vi "App - analyze RUS V6.vi"() -> ()   [LabVIEW 2018] (continued)
"last mod"=timestamp(3493887848 s since 1904-01-01), "file name str"="D:\\Data\\Ultrasound\\LSCO\\LSCO22__130814c\\5_Cooling_2nd_try\\September_2014\\091814\\14.54900K_500_2500_2.10000V_0.00000T_Sep18-2014__08-24-08_001_091814.bin", "mod time(min)"=58231464.13333333, "file format"=enum."binary", "power(V)"=2.1, "Magn Field(T) "=0.0}, {"temperature"=14.546, "temperature str"="14.54600", "file path"=path "D:/Data/Ultrasound/LSCO/LSCO22__130814c/5_Cooling_2nd_try/September_2014/091814/14.54600K_500_2500_2.10000V_0.00000T_Sep18-2014__08-25-27_001_091814.bin", "last mod"=timestamp(3493887927 s since 1904-01-01), "file name str"="D:\\Data\\Ultrasound\\LSCO\\LSCO22__130814c\\5_Cooling_2nd_try\\September_2014\\091814\\14.54600K_500_2500_2.10000V_0.00000T_Sep18-2014__08-25-27_001_091814.bin", "mod time(min)"=58231465.45, "file format"=enum."binary", "power(V)"=2.1, "Magn Field(T) "=0.0}, {"temperature"=14.55, "temperature str"="14.55000", "file path"=path "D:/Data/Ultrasound/LSCO/LSCO22__130814c/5_Cooling_2nd_try/September_2014/091814/14.55000K_500_2500_2.10000V_0.00000T_Sep18-2014__08-26-47_001_091814.bin", "last mod"=timestamp(3493888007 s since 1904-01-01), "file name str"="D:\\Data\\Ultrasound\\LSCO\\LSCO22__130814c\\5_Cooling_2nd_try\\September_2014\\091814\\14.55000K_500_2500_2.10000V_0.00000T_Sep18-2014__08-26-47_001_091814.bin", "mod time(min)"=58231466.78333333, "file format"=enum."binary", "power(V)"=2.1, "Magn Field(T) "=0.0}, {"temperature"=14.556, "temperature str"="14.55600", "file path"=path "D:/Data/Ultrasound/LSCO/LSCO22__130814c/5_Cooling_2nd_try/September_2014/091814/14.55600K_500_2500_2.10000V_0.00000T_Sep18-2014__08-28-06_001_091814.bin", "last mod"=timestamp(3493888086 s since 1904-01-01), "file name str"="D:\\Data\\Ultrasound\\LSCO\\LSCO22__130814c\\5_Cooling_2nd_try\\September_2014\\091814\\14.55600K_500_2500_2.10000V_0.00000T_Sep18-2014__08-28-06_001_091814.bin", "mod time(min)"=58231468.1, "file format"=enum."binary", "power(V)"=2.1, "Magn Field(T) "=0.0}, {"temperature"=14.554, "temperature str"="14.55400", "file path"=path "D:/Data/Ultrasound/LSCO/LSCO22__130814c/5_Cooling_2nd_try/September_2014/091814/14.55400K_500_2500_2.10000V_0.00000T_Sep18-2014__08-29-25_001_091814.bin", "last mod"=timestamp(3493888165 s since 1904-01-01), "file name str"="D:\\Data\\Ultrasound\\LSCO\\LSCO22__130814c\\5_Cooling_2nd_try\\September_2014\\091814\\14.55400K_500_2500_2.10000V_0.00000T_Sep18-2014__08-29-25_001_091814.bin", "mod time(min)"=58231469.416666664, "file format"=enum."binary", "power(V)"=2.1, "Magn Field(T) "=0.0}, {"temperature"=14.553, "temperature str"="14.55300", "file path"=path "D:/Data/Ultrasound/LSCO/LSCO22__130814c/5_Cooling_2nd_try/September_2014/091814/14.55300K_500_2500_2.10000V_0.00000T_Sep18-2014__08-30-45_001_091814.bin", "last mod"=timestamp(3493888245 s since 1904-01-01), "file name str"="D:\\Data\\Ultrasound\\LSCO\\LSCO22__130814c\\5_Cooling_2nd_try\\September_2014\\091814\\14.55300K_500_2500_2.10000V_0.00000T_Sep18-2014__08-30-45_001_091814.bin", "mod time(min)"=58231470.75, "file format"=enum."binary", "power(V)"=2.1, "Magn Field(T) "=0.0}, {"temperature"=14.556, "temperature str"="14.55600", "file path"=path "D:/Data/Ultrasound/LSCO/LSCO22__130814c/5_Cooling_2nd_try/September_2014/091814/14.55600K_500_2500_2.10000V_0.00000T_Sep18-2014__08-32-04_001_091814.bin", "last mod"=timestamp(3493888324 s since 1904-01-01), "file name str"="D:\\Data\\Ultrasound\\LSCO\\LSCO22__130814c\\5_Cooling_2nd_try\\September_2014\\091814\\14.55600K_500_2500_2.10000V_0.00000T_Sep18-2014__08-32-04_001_091814.bin", "mod time(min)"=58231472.06666667, "file format"=enum."binary", "power(V)"=2.1, "Magn Field(T) "=0.0}, {"temperature"=14.556, "temperature str"="14.55600", "file path"=path "D:/Data/Ultrasound/LSCO/LSCO22__130814c/5_Cooling_2nd_try/September_2014/091814/14.55600K_500_2500_2.10000V_0.00000T_Sep18-2014__08-33-24_001_091814.bin", "last mod"=timestamp(3493888404 s since 1904-01-01), "file name str"="D:\\Data\\Ultrasound\\LSCO\\LSCO22__130814c\\5_Cooling_2nd_try\\September_2014\\091814\\14.55600K_500_2500_2.10000V_0.00000T_Sep18-2014__08-33-24_001_091814.bin", "mod time(min)"=58231473.4, "file format"=enum."binary", "power(V)"=2.1, "Magn Field(T) "=0.0}, {"temperature"=14.56, "temperature str"="14.56000", "file path"=path "D:/Data/Ultrasound/LSCO/LSCO22__130814c/5_Cooling_2nd_try/September_2014/091814/14.56000K_500_2500_2.10000V_0.00000T_Sep18-2014__08-34-43_001_091814.bin", "last mod"=timestamp(3493888483 s since 1904-01-01), "file name str"="D:\\Data\\Ultrasound\\LSCO\\LSCO22__130814c\\5_Cooling_2nd_try\\September_2014\\091814\\14.56000K_500_2500_2.10000V_0.00000T_Sep18-2014__08-34-43_001_091814.bin", "mod time(min)"=58231474.71666667, "file format"=enum."binary", "power(V)"=2.1, "Magn Field(T) "=0.0}, {"temperature"=14.56, "temperature str"="14.56000", "file path"=path "D:/Data/Ultrasound/LSCO/LSCO22__130814c/5_Cooling_2nd_try/September_2014/091814/14.56000K_500_2500_2.10000V_0.00000T_Sep18-2014__08-36-02_001_091814.bin", "last mod"=timestamp(3493888562 s since 1904-01-01), "file name str"="D:\\Data\\Ultrasound\\LSCO\\LSCO22__130814c\\5_Cooling_2nd_try\\September_2014\\091814\\14.56000K_500_2500_2.10000V_0.00000T_Sep18-2014__08-36-02_001_091814.bin", "mod time(min)"=58231476.03333333, "file format"=enum."binary", "power(V)"=2.1, "Magn Field(T) "=0.0}, {"temperature"=14.561, "temperature str"="14.56100", "file path"=path "D:/Data/Ultrasound/LSCO/LSCO22__130814c/5_Cooling_2nd_try/September_2014/091814/14.56100K_500_2500_2.10000V_0.00000T_Sep18-2014__08-37-22_001_091814.bin", "last mod"=timestamp(3493888642 s since 1904-01-01), "file name str"="D:\\Data\\Ultrasound\\LSCO\\LSCO22__130814c\\5_Cooling_2nd_try\\September_2014\\091814\\14.56100K_500_2500_2.10000V_0.00000T_Sep18-2014__08-37-22_001_091814.bin", "mod time(min)"=58231477.36666667, "file format"=enum."binary", "power(V)"=2.1, "Magn Field(T) "=0.0}, {"temperature"=14.562, "temperature str"="14.56200", "file path"=path "D:/Data/Ultrasound/LSCO/LSCO22__130814c/5_Cooling_2nd_try/September_2014/091814/14.56200K_500_2500_2.10000V_0.00000T_Sep18-2014__08-38-41_001_091814.bin", "last mod"=timestamp(3493888721 s since 1904-01-01), "file name str"="D:\\Data\\Ultrasound\\LSCO\\LSCO22__130814c\\5_Cooling_2nd_try\\September_2014\\091814\\14.56200K_500_2500_2.10000V_0.00000T_Sep18-2014__08-38-41_001_091814.bin", "mod time(min)"=58231478.68333333, "file format"=enum."binary", "power(V)"=2.1, "Magn Field(T) "=0.0}, {"temperature"=14.56, "temperature str"="14.56000", "file path"=path "D:/Data/Ultrasound/LSCO/LSCO22__130814c/5_Cooling_2nd_try/September_2014/091814/14.56000K_500_2500_2.10000V_0.00000T_Sep18-2014__08-40-00_001_091814.bin", "last mod"=timestamp(3493888800 s since 1904-01-01), "file name str"="D:\\Data\\Ultrasound\\LSCO\\LSCO22__130814c\\5_Cooling_2nd_try\\September_2014\\091814\\14.56000K_500_2500_2.10000V_0.00000T_Sep18-2014__08-40-00_001_091814.bin", "mod time(min)"=58231480.0, "file format"=enum."binary", "power(V)"=2.1, "Magn Field(T) "=0.0}, {"temperature"=14.56, "temperature str"="14.56000", "file path"=path "D:/Data/Ultrasound/LSCO/LSCO22__130814c/5_Cooling_2nd_try/September_2014/091814/14.56000K_500_2500_2.10000V_0.00000T_Sep18-2014__08-41-20_001_091814.bin", "last mod"=timestamp(3493888880 s since 1904-01-01), "file name str"="D:\\Data\\Ultrasound\\LSCO\\LSCO22__130814c\\5_Cooling_2nd_try\\September_2014\\091814\\14.56000K_500_2500_2.10000V_0.00000T_Sep18-2014__08-41-20_001_091814.bin", "mod time(min)"=58231481.333333336, "file format"=enum."binary", "power(V)"=2.1, "Magn Field(T) "=0.0}, {"temperature"=14.561, "temperature str"="14.56100", "file path"=path "D:/Data/Ultrasound/LSCO/LSCO22__130814c/5_Cooling_2nd_try/September_2014/091814/14.56100K_500_2500_2.10000V_0.00000T_Sep18-2014__08-42-39_001_091814.bin", "last mod"=timestamp(3493888959 s since 1904-01-01), "file name str"="D:\\Data\\Ultrasound\\LSCO\\LSCO22__130814c\\5_Cooling_2nd_try\\September_2014\\091814\\14.56100K_500_2500_2.10000V_0.00000T_Sep18-2014__08-42-39_001_091814.bin", "mod time(min)"=58231482.65, "file format"=enum."binary", "power(V)"=2.1, "Magn Field(T) "=0.0}, {"temperature"=14.563, "temperature str"="14.56300", "file path"=path "D:/Data/Ultrasound/LSCO/LSCO22__130814c/5_Cooling_2nd_try/September_2014/091814/14.56300K_500_2500_2.10000V_0.00000T_Sep18-2014__08-43-59_001_091814.bin", "last mod"=timestamp(3493889039 s since 1904-01-01), "file name str"="D:\\Data\\Ultrasound\\LSCO\\LSCO22__130814c\\5_Cooling_2nd_try\\September_2014\\091814\\14.56300K_500_2500_2.10000V_0.00000T_Sep18-2014__08-43-59_001_091814.bin", "mod time(min)"=58231483.983333334, "file format"=enum."binary", "power(V)"=2.1, "Magn Field(T) "=0.0}, {"temperature"=14.564, "temperature str"="14.56400", "file path"=path "D:/Data/Ultrasound/LSCO/LSCO22__130814c/5_Cooling_2nd_try/September_2014/091814/14.56400K_500_2500_2.10000V_0.00000T_Sep18-2014__08-45-18_001_091814.bin", "last mod"=timestamp(3493889118 s since 1904-01-01), "file name str"="D:\\Data\\Ultrasound\\LSCO\\LSCO22__130814c\\5_Cooling_2nd_try\\September_2014\\091814\\14.56400K_500_2500_2.10000V_0.00000T_Sep18-2014__08-45-18_001_091814.bin", "mod time(min)"=58231485.3, "file format"=enum."binary", "power(V)"=2.1, "Magn Field(T) "=0.0}, {"temperature"=14.572, "temperature str"="14.57200", "file path"=path "D:/Data/Ultrasound/LSCO/LSCO22__130814c/5_Cooling_2nd_try/September_2014/091814/14.57200K_500_2500_2.10000V_0.00000T_Sep18-2014__08-46-37_001_091814.bin", "last mod"=timestamp(3493889197 s since 1904-01-01), "file name str"="D:\\Data\\Ultrasound\\LSCO\\LSCO22__130814c\\5_Cooling_2nd_try\\September_2014\\091814\\14.57200K_500_2500_2.10000V_0.00000T_Sep18-2014__08-46-37_001_091814.bin", "mod time(min)"=58231486.61666667, "file format"=enum."binary", "power(V)"=2.1, "Magn Field(T) "=0.0}, {"temperature"=14.568, "temperature str"="14.56800", "file path"=path "D:/Data/Ultrasound/LSCO/LSCO22__130814c/5_Cooling_2nd_try/September_2014/091814/14.56800K_500_2500_2.10000V_0.00000T_Sep18-2014__08-47-57_001_091814.bin", "last mod"=timestamp(3493889277 s since 1904-01-01), "file name str"="D:\\Data\\Ultrasound\\LSCO\\LSCO22__130814c\\5_Cooling_2nd_try\\September_2014\\091814\\14.56800K_500_2500_2.10000V_0.00000T_Sep18-2014__08-47-57_001_091814.bin", "mod time(min)"=58231487.95, "file format"=enum."binary", "power(V)"=2.1, "Magn Field(T) "=0.0}, {"temperature"=14.565, "temperature str"="14.56500", "file path"=path "D:/Data/Ultrasound/LSCO/LSCO22__130814c/5_Cooling_2nd_try/September_2014/091814/14.56500K_500_2500_2.10000V_0.00000T_Sep18-2014__08-49-16_001_091814.bin", "last mod"=timestamp(3493889356 s since 1904-01-01), "file name str"="D:\\Data\\Ultrasound\\LSCO\\LSCO22__130814c\\5_Cooling_2nd_try\\September_2014\\091814\\14.56500K_500_2500_2.10000V_0.00000T_Sep18-2014__08-49-16_001_091814.bin", "mod time(min)"=58231489.266666666, "file format"=enum."binary", "power(V)"=2.1, "Magn Field(T) "=0.0}, {"temperature"=14.569, "temperature str"="14.56900", "file path"=path "D:/Data/Ultrasound/LSCO/LSCO22__130814c/5_Cooling_2nd_try/September_2014/091814/14.56900K_500_2500_2.10000V_0.00000T_Sep18-2014__08-50-36_001_091814.bin", "last mod"=timestamp(3493889436 s since 1904-01-01), "file name str"="D:\\Data\\Ultrasound\\LSCO\\LSCO22__130814c\\5_Cooling_2nd_try\\September_2014\\091814\\14.56900K_500_2500_2.10000V_0.00000T_Sep18-2014__08-50-36_001_091814.bin", "mod time(min)"=58231490.6, "file format"=enum."binary", "power(V)"=2.1, "Magn Field(T) "=0.0}, {"temperature"=14.577, "temperature str"="14.57700", "file path"=path "D:/Data/Ultrasound/LSCO/LSCO22__130814c/5_Cooling_2nd_try/September_2014/091814/14.57700K_500_2500_2.10000V_0.00000T_Sep18-2014__08-51-55_001_091814.bin", "last mod"=timestamp(3493889515 s since 1904-01-01), "file name str"="D:\\Data\\Ultrasound\\LSCO\\LSCO22__130814c\\5_Cooling_2nd_try\\September_2014\\091814\\14.57700K_500_2500_2.10000V_0.00000T_Sep18-2014__08-51-55_001_091814.bin", "mod time(min)"=58231491.916666664, "file format"=enum."binary", "power(V)"=2.1, "Magn Field(T) "=0.0}, {"temperature"=14.571, "temperature str"="14.57100", "file path"=path "D:/Data/Ultrasound/LSCO/LSCO22__130814c/5_Cooling_2nd_try/September_2014/091814/14.57100K_500_2500_2.10000V_0.00000T_Sep18-2014__08-53-14_001_091814.bin", "last mod"=timestamp(3493889594 s since 1904-01-01), "file name str"="D:\\Data\\Ultrasound\\LSCO\\LSCO22__130814c\\5_Cooling_2nd_try\\September_2014\\091814\\14.57100K_500_2500_2.10000V_0.00000T_Sep18-2014__08-53-14_001_091814.bin", "mod time(min)"=58231493.233333334, "file format"=enum."binary", "power(V)"=2.1, "Magn Field(T) "=0.0}, {"temperature"=14.58, "temperature str"="14.58000", "file path"=path "D:/Data/Ultrasound/LSCO/LSCO22__130814c/5_Cooling_2nd_try/September_2014/091814/14.58000K_500_2500_2.10000V_0.00000T_Sep18-2014__08-54-34_001_091814.bin", "last mod"=timestamp(3493889674 s since 1904-01-01), "file name str"="D:\\Data\\Ultrasound\\LSCO\\LSCO22__130814c\\5_Cooling_2nd_try\\September_2014\\091814\\14.58000K_500_2500_2.10000V_0.00000T_Sep18-2014__08-54-34_001_091814.bin", "mod time(min)"=58231494.56666667, "file format"=enum."binary", "power(V)"=2.1, "Magn Field(T) "=0.0}, {"temperature"=14.578, "temperature str"="14.57800", "file path"=path "D:/Data/Ultrasound/LSCO/LSCO22__130814c/5_Cooling_2nd_try/September_2014/091814/14.57800K_500_2500_2.10000V_0.00000T_Sep18-2014__08-55-53_001_091814.bin", "last mod"=timestamp(3493889753 s since 1904-01-01), "file name str"="D:\\Data\\Ultrasound\\LSCO\\LSCO22__130814c\\5_Cooling_2nd_try\\September_2014\\091814\\14.57800K_500_2500_2.10000V_0.00000T_Sep18-2014__08-55-53_001_091814.bin", "mod time(min)"=58231495.88333333, "file format"=enum."binary", "power(V)"=2.1, "Magn Field(T) "=0.0}, {"temperature"=14.579, "temperature str"="14.57900", "file path"=path "D:/Data/Ultrasound/LSCO/LSCO22__130814c/5_Cooling_2nd_try/September_2014/091814/14.57900K_500_2500_2.10000V_0.00000T_Sep18-2014__08-57-12_001_091814.bin", "last mod"=timestamp(3493889832 s since 1904-01-01), "file name str"="D:\\Data\\Ultrasound\\LSCO\\LSCO22__130814c\\5_Cooling_2nd_try\\September_2014\\091814\\14.57900K_500_2500_2.10000V_0.00000T_Sep18-2014__08-57-12_001_091814.bin", "mod time(min)"=58231497.2, "file format"=enum."binary", "power(V)"=2.1, "Magn Field(T) "=0.0}, {"temperature"=14.581, "temperature str"="14.58100", "file path"=path "D:/Data/Ultrasound/LSCO/LSCO22__130814c/5_Cooling_2nd_try/September_2014/091814/14.58100K_500_2500_2.10000V_0.00000T_Sep18-2014__08-58-31_001_091814.bin", "last mod"=timestamp(3493889911 s since 1904-01-01), "file name str"="D:\\Data\\Ultrasound\\LSCO\\LSCO22__130814c\\5_Cooling_2nd_try\\September_2014\\091814\\14.58100K_500_2500_2.10000V_0.00000T_Sep18-2014__08-58-31_001_091814.bin", "mod time(min)"=58231498.516666666, "file format"=enum."binary", "power(V)"=2.1, "Magn Field(T) "=0.0}, {"temperature"=14.58, "temperature str"="14.58000", "file path"=path "D:/Data/Ultrasound/LSCO/LSCO22__130814c/5_Cooling_2nd_try/September_2014/091814/14.58000K_500_2500_2.10000V_0.00000T_Sep18-2014__08-59-50_001_091814.bin", "last mod"=timestamp(3493889990 s since 1904-01-01), "file name str"="D:\\Data\\Ultrasound\\LSCO\\LSCO22__130814c\\5_Cooling_2nd_try\\September_2014\\091814\\14.58000K_500_2500_2.10000V_0.00000T_Sep18-2014__08-59-50_001_091814.bin", "mod time(min)"=58231499.833333336, "file format"=enum."binary", "power(V)"=2.1, "Magn Field(T) "=0.0}, {"temperature"=14.577, "temperature str"="14.57700", "file path"=path "D:/Data/Ultrasound/LSCO/LSCO22__130814c/5_Cooling_2nd_try/September_2014/091814/14.57700K_500_2500_2.10000V_0.00000T_Sep18-2014__09-01-10_001_091814.bin", "last mod"=timestamp(3493890070 s since 1904-01-01), "file name str"="D:\\Data\\Ultrasound\\LSCO\\LSCO22__130814c\\5_Cooling_2nd_try\\September_2014\\091814\\14.57700K_500_2500_2.10000V_0.00000T_Sep18-2014__09-01-10_001_091814.bin", "mod time(min)"=58231501.166666664, "file format"=enum."binary", "power(V)"=2.1, "Magn Field(T) "=0.0}, {"temperature"=14.58, "temperature str"="14.58000", "file path"=path "D:/Data/Ultrasound/LSCO/LSCO22__130814c/5_Cooling_2nd_try/September_2014/091814/14.58000K_500_2500_2.10000V_0.00000T_Sep18-2014__09-02-29_001_091814.bin", "last mod"=timestamp(3493890149 s since 1904-01-01), "file name str"="D:\\Data\\Ultrasound\\LSCO\\LSCO22__130814c\\5_Cooling_2nd_try\\September_2014\\091814\\14.58000K_500_2500_2.10000V_0.00000T_Sep18-2014__09-02-29_001_091814.bin", "mod time(min)"=58231502.483333334, "file format"=enum."binary", "power(V)"=2.1, "Magn Field(T) "=0.0}, {"temperature"=14.583, "temperature str"="14.58300", "file path"=path "D:/Data/Ultrasound/LSCO/LSCO22__130814c/5_Cooling_2nd_try/September_2014/091814/14.58300K_500_2500_2.10000V_0.00000T_Sep18-2014__09-03-48_001_091814.bin", "last mod"=timestamp(3493890228 s since 1904-01-01), "file name str"="D:\\Data\\Ultrasound\\LSCO\\LSCO22__130814c\\5_Cooling_2nd_try\\September_2014\\091814\\14.58300K_500_2500_2.10000V_0.00000T_Sep18-2014__09-03-48_001_091814.bin", "mod time(min)"=58231503.8, "file format"=enum."binary", "power(V)"=2.1, "Magn Field(T) "=0.0}, {"temperature"=14.582, "temperature str"="14.58200", "file path"=path "D:/Data/Ultrasound/LSCO/LSCO22__130814c/5_Cooling_2nd_try/September_2014/091814/14.58200K_500_2500_2.10000V_0.00000T_Sep18-2014__09-05-08_001_091814.bin", "last mod"=timestamp(3493890308 s since 1904-01-01), "file name str"="D:\\Data\\Ultrasound\\LSCO\\LSCO22__130814c\\5_Cooling_2nd_try\\September_2014\\091814\\14.58200K_500_2500_2.10000V_0.00000T_Sep18-2014__09-05-08_001_091814.bin", "mod time(min)"=58231505.13333333, "file format"=enum."binary", "power(V)"=2.1, "Magn Field(T) "=0.0}, {"temperature"=14.584, "temperature str"="14.58400", "file path"=path "D:/Data/Ultrasound/LSCO/LSCO22__130814c/5_Cooling_2nd_try/September_2014/091814/14.58400K_500_2500_2.10000V_0.00000T_Sep18-2014__09-06-27_001_091814.bin", "last mod"=timestamp(3493890387 s since 1904-01-01), "file name str"="D:\\Data\\Ultrasound\\LSCO\\LSCO22__130814c\\5_Cooling_2nd_try\\September_2014\\091814\\14.58400K_500_2500_2.10000V_0.00000T_Sep18-2014__09-06-27_001_091814.bin", "mod time(min)"=58231506.45, "file format"=enum."binary", "power(V)"=2.1, "Magn Field(T) "=0.0}, {"temperature"=14.584, "temperature str"="14.58400", "file path"=path "D:/Data/Ultrasound/LSCO/LSCO22__130814c/5_Cooling_2nd_try/September_2014/091814/14.58400K_500_2500_2.10000V_0.00000T_Sep18-2014__09-07-46_001_091814.bin", "last mod"=timestamp(3493890466 s since 1904-01-01), "file name str"="D:\\Data\\Ultrasound\\LSCO\\LSCO22__130814c\\5_Cooling_2nd_try\\September_2014\\091814\\14.58400K_500_2500_2.10000V_0.00000T_Sep18-2014__09-07-46_001_091814.bin", "mod time(min)"=58231507.766666666, "file format"=enum."binary", "power(V)"=2.1, "Magn Field(T) "=0.0}, {"temperature"=14.585, "temperature str"="14.58500", "file path"=path "D:/Data/Ultrasound/LSCO/LSCO22__130814c/5_Cooling_2nd_try/September_2014/091814/14.58500K_500_2500_2.10000V_0.00000T_Sep18-2014__09-09-06_001_091814.bin", "last mod"=timestamp(3493890546 s since 1904-01-01), "file name str"="D:\\Data\\Ultrasound\\LSCO\\LSCO22__130814c\\5_Cooling_2nd_try\\September_2014\\091814\\14.58500K_500_2500_2.10000V_0.00000T_Sep18-2014__09-09-06_001_091814.bin", "mod time(min)"=58231509.1, "file format"=enum."binary", "power(V)"=2.1, "Magn Field(T) "=0.0}, {"temperature"=14.585, "temperature str"="14.58500", "file path"=path "D:/Data/Ultrasound/LSCO/LSCO22__130814c/5_Cooling_2nd_try/September_2014/091814/14.58500K_500_2500_2.10000V_0.00000T_Sep18-2014__09-10-25_001_091814.bin", "last mod"=timestamp(3493890625 s since 1904-01-01), "file name str"="D:\\Data\\Ultrasound\\LSCO\\LSCO22__130814c\\5_Cooling_2nd_try\\September_2014\\091814\\14.58500K_500_2500_2.10000V_0.00000T_Sep18-2014__09-10-25_001_091814.bin", "mod time(min)"=58231510.416666664, "file format"=enum."binary", "power(V)"=2.1, "Magn Field(T) "=0.0}, {"temperature"=14.585, "temperature str"="14.58500", "file path"=path "D:/Data/Ultrasound/LSCO/LSCO22__130814c/5_Cooling_2nd_try/September_2014/091814/14.58500K_500_2500_2.10000V_0.00000T_Sep18-2014__09-11-44_001_091814.bin", "last mod"=timestamp(3493890704 s since 1904-01-01), "file name str"="D:\\Data\\Ultrasound\\LSCO\\LSCO22__130814c\\5_Cooling_2nd_try\\September_2014\\091814\\14.58500K_500_2500_2.10000V_0.00000T_Sep18-2014__09-11-44_001_091814.bin", "mod time(min)"=58231511.733333334, "file format"=enum."binary", "power(V)"=2.1, "Magn Field(T) "=0.0}, {"temperature"=14.585, "temperature str"="14.58500", "file path"=path "D:/Data/Ultrasound/LSCO/LSCO22__130814c/5_Cooling_2nd_try/September_2014/091814/14.58500K_500_2500_2.10000V_0.00000T_Sep18-2014__09-13-04_001_091814.bin", "last mod"=timestamp(3493890784 s since 1904-01-01), "file name str"="D:\\Data\\Ultrasound\\LSCO\\LSCO22__130814c\\5_Cooling_2nd_try\\September_2014\\091814\\14.58500K_500_2500_2.10000V_0.00000T_Sep18-2014__09-13-04_001_091814.bin", "mod time(min)"=58231513.06666667, "file format"=enum."binary", "power(V)"=2.1, "Magn Field(T) "=0.0}, {"temperature"=14.587, "temperature str"="14.58700", "file path"=path "D:/Data/Ultrasound/LSCO/LSCO22__130814c/5_Cooling_2nd_try/September_2014/091814/14.58700K_500_2500_2.10000V_0.00000T_Sep18-2014__09-14-23_001_091814.bin", "last mod"=timestamp(3493890863 s since 1904-01-01), "file name str"="D:\\Data\\Ultrasound\\LSCO\\LSCO22__130814c\\5_Cooling_2nd_try\\September_2014\\091814\\14.58700K_500_2500_2.10000V_0.00000T_Sep18-2014__09-14-23_001_091814.bin", "mod time(min)"=58231514.38333333, "file format"=enum."binary", "power(V)"=2.1, "Magn Field(T) "=0.0}, {"temperature"=14.593, "temperature str"="14.59300", "file path"=path "D:/Data/Ultrasound/LSCO/LSCO22__130814c/5_Cooling_2nd_try/September_2014/091814/14.59300K_500_2500_2.10000V_0.00000T_Sep18-2014__09-15-43_001_091814.bin", "last mod"=timestamp(3493890943 s since 1904-01-01), "file name str"="D:\\Data\\Ultrasound\\LSCO\\LSCO22__130814c\\5_Cooling_2nd_try\\September_2014\\091814\\14.59300K_500_2500_2.10000V_0.00000T_Sep18-2014__09-15-43_001_091814.bin", "mod time(min)"=58231515.71666667, "file format"=enum."binary", "power(V)"=2.1, "Magn Field(T) "=0.0}, {"temperature"=14.595, "temperature str"="14.59500", "file path"=path "D:/Data/Ultrasound/LSCO/LSCO22__130814c/5_Cooling_2nd_try/September_2014/091814/14.59500K_500_2500_2.10000V_0.00000T_Sep18-2014__09-17-02_001_091814.bin", "last mod"=timestamp(3493891022 s since 1904-01-01), "file name str"="D:\\Data\\Ultrasound\\LSCO\\LSCO22__130814c\\5_Cooling_2nd_try\\September_2014\\091814\\14.59500K_500_2500_2.10000V_0.00000T_Sep18-2014__09-17-02_001_091814.bin", "mod time(min)"=58231517.03333333, "file format"=enum."binary", "power(V)"=2.1, "Magn Field(T) "=0.0}, {"temperature"=14.597, "temperature str"="14.59700", "file path"=path "D:/Data/Ultrasound/LSCO/LSCO22__130814c/5_Cooling_2nd_try/September_2014/091814/14.59700K_500_2500_2.10000V_0.00000T_Sep18-2014__09-18-21_001_091814.bin", "last mod"=timestamp(3493891101 s since 1904-01-01), "file name str"="D:\\Data\\Ultrasound\\LSCO\\LSCO22__130814c\\5_Cooling_2nd_try\\September_2014\\091814\\14.59700K_500_2500_2.10000V_0.00000T_Sep18-2014__09-18-21_001_091814.bin", "mod time(min)"=58231518.35, "file format"=enum."binary", "power(V)"=2.1, "Magn Field(T) "=0.0}, {"temperature"=14.595, "temperature str"="14.59500", "file path"=path "D:/Data/Ultrasound/LSCO/LSCO22__130814c/5_Cooling_2nd_try/September_2014/091814/14.59500K_500_2500_2.10000V_0.00000T_Sep18-2014__09-19-41_001_091814.bin", "last mod"=timestamp(3493891181 s since 1904-01-01), "file name str"="D:\\Data\\Ultrasound\\LSCO\\LSCO22__130814c\\5_Cooling_2nd_try\\September_2014\\091814\\14.59500K_500_2500_2.10000V_0.00000T_Sep18-2014__09-19-41_001_091814.bin", "mod time(min)"=58231519.68333333, "file format"=enum."binary", "power(V)"=2.1, "Magn Field(T) "=0.0}, {"temperature"=14.597, "temperature str"="14.59700", "file path"=path "D:/Data/Ultrasound/LSCO/LSCO22__130814c/5_Cooling_2nd_try/September_2014/091814/14.59700K_500_2500_2.10000V_0.00000T_Sep18-2014__09-21-00_001_091814.bin", "last mod"=timestamp(3493891260 s since 1904-01-01), "file name str"="D:\\Data\\Ultrasound\\LSCO\\LSCO22__130814c\\5_Cooling_2nd_try\\September_2014\\091814\\14.59700K_500_2500_2.10000V_0.00000T_Sep18-2014__09-21-00_001_091814.bin", "mod time(min)"=58231521.0, "file format"=enum."binary", "power(V)"=2.1, "Magn Field(T) "=0.0}, {"temperature"=14.595, "temperature str"="14.59500", "file path"=path "D:/Data/Ultrasound/LSCO/LSCO22__130814c/5_Cooling_2nd_try/September_2014/091814/14.59500K_500_2500_2.10000V_0.00000T_Sep18-2014__09-22-19_001_091814.bin", "last mod"=timestamp(3493891339 s since 1904-01-01), "file name str"="D:\\Data\\Ultrasound\\LSCO\\LSCO22__130814c\\5_Cooling_2nd_try\\September_2014\\091814\\14.59500K_500_2500_2.10000V_0.00000T_Sep18-2014__09-22-19_001_091814.bin", "mod time(min)"=58231522.31666667, "file format"=enum."binary", "power(V)"=2.1, "Magn Field(T) "=0.0}, {"temperature"=14.597, "temperature str"="14.59700", "file path"=path "D:/Data/Ultrasound/LSCO/LSCO22__130814c/5_Cooling_2nd_try/September_2014/091814/14.59700K_500_2500_2.10000V_0.00000T_Sep18-2014__09-23-39_001_091814.bin", "last mod"=timestamp(3493891419 s since 1904-01-01), "file name str"="D:\\Data\\Ultrasound\\LSCO\\LSCO22__130814c\\5_Cooling_2nd_try\\September_2014\\091814\\14.59700K_500_2500_2.10000V_0.00000T_Sep18-2014__09-23-39_001_091814.bin", "mod time(min)"=58231523.65, "file format"=enum."binary", "power(V)"=2.1, "Magn Field(T) "=0.0}, {"temperature"=14.597, "temperature str"="14.59700", "file path"=path "D:/Data/Ultrasound/LSCO/LSCO22__130814c/5_Cooling_2nd_try/September_2014/091814/14.59700K_500_2500_2.10000V_0.00000T_Sep18-2014__09-24-58_001_091814.bin", "last mod"=timestamp(3493891498 s since 1904-01-01), "file name str"="D:\\Data\\Ultrasound\\LSCO\\LSCO22__130814c\\5_Cooling_2nd_try\\September_2014\\091814\\14.59700K_500_2500_2.10000V_0.00000T_Sep18-2014__09-24-58_001_091814.bin", "mod time(min)"=58231524.96666667, "file format"=enum."binary", "power(V)"=2.1, "Magn Field(T) "=0.0}, {"temperature"=14.599, "temperature str"="14.59900", "file path"=path "D:/Data/Ultrasound/LSCO/LSCO22__130814c/5_Cooling_2nd_try/September_2014/091814/14.59900K_500_2500_2.10000V_0.00000T_Sep18-2014__09-26-18_001_091814.bin", "last mod"=timestamp(3493891578 s since 1904-01-01), "file name str"="D:\\Data\\Ultrasound\\LSCO\\LSCO22__130814c\\5_Cooling_2nd_try\\September_2014\\091814\\14.59900K_500_2500_2.10000V_0.00000T_Sep18-2014__09-26-18_001_091814.bin", "mod time(min)"=58231526.3, "file format"=enum."binary", "power(V)"=2.1, "Magn Field(T) "=0.0}, {"temperature"=14.599, "temperature str"="14.59900", "file path"=path "D:/Data/Ultrasound/LSCO/LSCO22__130814c/5_Cooling_2nd_try/September_2014/091814/14.59900K_500_2500_2.10000V_0.00000T_Sep18-2014__09-27-37_001_091814.bin", "last mod"=timestamp(3493891657 s since 1904-01-01), "file name str"="D:\\Data\\Ultrasound\\LSCO\\LSCO22__130814c\\5_Cooling_2nd_try\\September_2014\\091814\\14.59900K_500_2500_2.10000V_0.00000T_Sep18-2014__09-27-37_001_091814.bin", "mod time(min)"=58231527.61666667, "file format"=enum."binary", "power(V)"=2.1, "Magn Field(T) "=0.0}, {"temperature"=14.599, "temperature str"="14.59900", "file path"=path "D:/Data/Ultrasound/LSCO/LSCO22__130814c/5_Cooling_2nd_try/September_2014/091814/14.59900K_500_2500_2.10000V_0.00000T_Sep18-2014__09-28-56_001_091814.bin", "last mod"=timestamp(3493891736 s since 1904-01-01), "file name str"="D:\\Data\\Ultrasound\\LSCO\\LSCO22__130814c\\5_Cooling_2nd_try\\September_2014\\091814\\14.59900K_500_2500_2.10000V_0.00000T_Sep18-2014__09-28-56_001_091814.bin", "mod time(min)"=58231528.93333333, "file format"=enum."binary", "power(V)"=2.1, "Magn Field(T) "=0.0}, {"temperature"=14.601, "temperature str"="14.60100", "file path"=path "D:/Data/Ultrasound/LSCO/LSCO22__130814c/5_Cooling_2nd_try/September_2014/091814/14.60100K_500_2500_2.10000V_0.00000T_Sep18-2014__09-30-16_001_091814.bin", "last mod"=timestamp(3493891816 s since 1904-01-01), "file name str"="D:\\Data\\Ultrasound\\LSCO\\LSCO22__130814c\\5_Cooling_2nd_try\\September_2014\\091814\\14.60100K_500_2500_2.10000V_0.00000T_Sep18-2014__09-30-16_001_091814.bin", "mod time(min)"=58231530.266666666, "file format"=enum."binary", "power(V)"=2.1, "Magn Field(T) "=0.0}, {"temperature"=14.605, "temperature str"="14.60500", "file path"=path "D:/Data/Ultrasound/LSCO/LSCO22__130814c/5_Cooling_2nd_try/September_2014/091814/14.60500K_500_2500_2.10000V_0.00000T_Sep18-2014__09-31-35_001_091814.bin", "last mod"=timestamp(3493891895 s since 1904-01-01), "file name str"="D:\\Data\\Ultrasound\\LSCO\\LSCO22__130814c\\5_Cooling_2nd_try\\September_2014\\091814\\14.60500K_500_2500_2.10000V_0.00000T_Sep18-2014__09-31-35_001_091814.bin", "mod time(min)"=58231531.583333336, "file format"=enum."binary", "power(V)"=2.1, "Magn Field(T) "=0.0}, {"temperature"=14.604, "temperature str"="14.60400", "file path"=path "D:/Data/Ultrasound/LSCO/LSCO22__130814c/5_Cooling_2nd_try/September_2014/091814/14.60400K_500_2500_2.10000V_0.00000T_Sep18-2014__09-32-54_001_091814.bin", "last mod"=timestamp(3493891974 s since 1904-01-01), "file name str"="D:\\Data\\Ultrasound\\LSCO\\LSCO22__130814c\\5_Cooling_2nd_try\\September_2014\\091814\\14.60400K_500_2500_2.10000V_0.00000T_Sep18-2014__09-32-54_001_091814.bin", "mod time(min)"=58231532.9, "file format"=enum."binary", "power(V)"=2.1, "Magn Field(T) "=0.0}, {"temperature"=14.606, "temperature str"="14.60600", "file path"=path "D:/Data/Ultrasound/LSCO/LSCO22__130814c/5_Cooling_2nd_try/September_2014/091814/14.60600K_500_2500_2.10000V_0.00000T_Sep18-2014__09-34-14_001_091814.bin", "last mod"=timestamp(3493892054 s since 1904-01-01), "file name str"="D:\\Data\\Ultrasound\\LSCO\\LSCO22__130814c\\5_Cooling_2nd_try\\September_2014\\091814\\14.60600K_500_2500_2.10000V_0.00000T_Sep18-2014__09-34-14_001_091814.bin", "mod time(min)"=58231534.233333334, "file format"=enum."binary", "power(V)"=2.1, "Magn Field(T) "=0.0}, {"temperature"=14.606, "temperature str"="14.60600", "file path"=path "D:/Data/Ultrasound/LSCO/LSCO22__130814c/5_Cooling_2nd_try/September_2014/091814/14.60600K_500_2500_2.10000V_0.00000T_Sep18-2014__09-35-33_001_091814.bin", "last mod"=timestamp(3493892133 s since 1904-01-01), "file name str"="D:\\Data\\Ultrasound\\LSCO\\LSCO22__130814c\\5_Cooling_2nd_try\\September_2014\\091814\\14.60600K_500_2500_2.10000V_0.00000T_Sep18-2014__09-35-33_001_091814.bin", "mod time(min)"=58231535.55, "file format"=enum."binary", "power(V)"=2.1, "Magn Field(T) "=0.0}, {"temperature"=14.609, "temperature str"="14.60900", "file path"=path "D:/Data/Ultrasound/LSCO/LSCO22__130814c/5_Cooling_2nd_try/September_2014/091814/14.60900K_500_2500_2.10000V_0.00000T_Sep18-2014__09-36-53_001_091814.bin", "last mod"=timestamp(3493892213 s since 1904-01-01), "file name str"="D:\\Data\\Ultrasound\\LSCO\\LSCO22__130814c\\5_Cooling_2nd_try\\September_2014\\091814\\14.60900K_500_2500_2.10000V_0.00000T_Sep18-2014__09-36-53_001_091814.bin", "mod time(min)"=58231536.88333333, "file format"=enum."binary", "power(V)"=2.1, "Magn Field(T) "=0.0}, {"temperature"=14.613, "temperature str"="14.61300", "file path"=path "D:/Data/Ultrasound/LSCO/LSCO22__130814c/5_Cooling_2nd_try/September_2014/091814/14.61300K_500_2500_2.10000V_0.00000T_Sep18-2014__09-38-12_001_091814.bin", "last mod"=timestamp(3493892292 s since 1904-01-01), "file name str"="D:\\Data\\Ultrasound\\LSCO\\LSCO22__130814c\\5_Cooling_2nd_try\\September_2014\\091814\\14.61300K_500_2500_2.10000V_0.00000T_Sep18-2014__09-38-12_001_091814.bin", "mod time(min)"=58231538.2, "file format"=enum."binary", "power(V)"=2.1, "Magn Field(T) "=0.0}, {"temperature"=14.614, "temperature str"="14.61400", "file path"=path "D:/Data/Ultrasound/LSCO/LSCO22__130814c/5_Cooling_2nd_try/September_2014/091814/14.61400K_500_2500_2.10000V_0.00000T_Sep18-2014__09-39-31_001_091814.bin", "last mod"=timestamp(3493892371 s since 1904-01-01), "file name str"="D:\\Data\\Ultrasound\\LSCO\\LSCO22__130814c\\5_Cooling_2nd_try\\September_2014\\091814\\14.61400K_500_2500_2.10000V_0.00000T_Sep18-2014__09-39-31_001_091814.bin", "mod time(min)"=58231539.516666666, "file format"=enum."binary", "power(V)"=2.1, "Magn Field(T) "=0.0}, {"temperature"=14.619, "temperature str"="14.61900", "file path"=path "D:/Data/Ultrasound/LSCO/LSCO22__130814c/5_Cooling_2nd_try/September_2014/091814/14.61900K_500_2500_2.10000V_0.00000T_Sep18-2014__09-40-51_001_091814.bin", "last mod"=timestamp(3493892451 s since 1904-01-01), "file name str"="D:\\Data\\Ultrasound\\LSCO\\LSCO22__130814c\\5_Cooling_2nd_try\\September_2014\\091814\\14.61900K_500_2500_2.10000V_0.00000T_Sep18-2014__09-40-51_001_091814.bin", "mod time(min)"=58231540.85, "file format"=enum."binary", "power(V)"=2.1, "Magn Field(T) "=0.0}, {"temperature"=14.618, "temperature str"="14.61800", "file path"=path "D:/Data/Ultrasound/LSCO/LSCO22__130814c/5_Cooling_2nd_try/September_2014/091814/14.61800K_500_2500_2.10000V_0.00000T_Sep18-2014__09-42-10_001_091814.bin", "last mod"=timestamp(3493892530 s since 1904-01-01), "file name str"="D:\\Data\\Ultrasound\\LSCO\\LSCO22__130814c\\5_Cooling_2nd_try\\September_2014\\091814\\14.61800K_500_2500_2.10000V_0.00000T_Sep18-2014__09-42-10_001_091814.bin", "mod time(min)"=58231542.166666664, "file format"=enum."binary", "power(V)"=2.1, "Magn Field(T) "=0.0}, {"temperature"=14.62, "temperature str"="14.62000", "file path"=path "D:/Data/Ultrasound/LSCO/LSCO22__130814c/5_Cooling_2nd_try/September_2014/091814/14.62000K_500_2500_2.10000V_0.00000T_Sep18-2014__09-43-29_001_091814.bin", "last mod"=timestamp(3493892609 s since 1904-01-01), "file name str"="D:\\Data\\Ultrasound\\LSCO\\LSCO22__130814c\\5_Cooling_2nd_try\\September_2014\\091814\\14.62000K_500_2500_2.10000V_0.00000T_Sep18-2014__09-43-29_001_091814.bin", "mod time(min)"=58231543.483333334, "file format"=enum."binary", "power(V)"=2.1, "Magn Field(T) "=0.0}, {"temperature"=14.621, "temperature str"="14.62100", "file path"=path "D:/Data/Ultrasound/LSCO/LSCO22__130814c/5_Cooling_2nd_try/September_2014/091814/14.62100K_500_2500_2.10000V_0.00000T_Sep18-2014__09-44-49_001_091814.bin", "last mod"=timestamp(3493892689 s since 1904-01-01), "file name str"="D:\\Data\\Ultrasound\\LSCO\\LSCO22__130814c\\5_Cooling_2nd_try\\September_2014\\091814\\14.62100K_500_2500_2.10000V_0.00000T_Sep18-2014__09-44-49_001_091814.bin", "mod time(min)"=58231544.81666667, "file format"=enum."binary", "power(V)"=2.1, "Magn Field(T) "=0.0}, {"temperature"=14.623, "temperature str"="14.62300", "file path"=path "D:/Data/Ultrasound/LSCO/LSCO22__130814c/5_Cooling_2nd_try/September_2014/091814/14.62300K_500_2500_2.10000V_0.00000T_Sep18-2014__09-46-08_001_091814.bin", "last mod"=timestamp(3493892768 s since 1904-01-01), "file name str"="D:\\Data\\Ultrasound\\LSCO\\LSCO22__130814c\\5_Cooling_2nd_try\\September_2014\\091814\\14.62300K_500_2500_2.10000V_0.00000T_Sep18-2014__09-46-08_001_091814.bin", "mod time(min)"=58231546.13333333, "file format"=enum."binary", "power(V)"=2.1, "Magn Field(T) "=0.0}, {"temperature"=14.624, "temperature str"="14.62400", "file path"=path "D:/Data/Ultrasound/LSCO/LSCO22__130814c/5_Cooling_2nd_try/September_2014/091814/14.62400K_500_2500_2.10000V_0.00000T_Sep18-2014__09-47-28_001_091814.bin", "last mod"=timestamp(3493892848 s since 1904-01-01), "file name str"="D:\\Data\\Ultrasound\\LSCO\\LSCO22__130814c\\5_Cooling_2nd_try\\September_2014\\091814\\14.62400K_500_2500_2.10000V_0.00000T_Sep18-2014__09-47-28_001_091814.bin", "mod time(min)"=58231547.46666667, "file format"=enum."binary", "power(V)"=2.1, "Magn Field(T) "=0.0}, {"temperature"=14.628, "temperature str"="14.62800", "file path"=path "D:/Data/Ultrasound/LSCO/LSCO22__130814c/5_Cooling_2nd_try/September_2014/091814/14.62800K_500_2500_2.10000V_0.00000T_Sep18-2014__09-48-47_001_091814.bin", "last mod"=timestamp(3493892927 s since 1904-01-01), "file name str"="D:\\Data\\Ultrasound\\LSCO\\LSCO22__130814c\\5_Cooling_2nd_try\\September_2014\\091814\\14.62800K_500_2500_2.10000V_0.00000T_Sep18-2014__09-48-47_001_091814.bin", "mod time(min)"=58231548.78333333, "file format"=enum."binary", "power(V)"=2.1, "Magn Field(T) "=0.0}, {"temperature"=14.625, "temperature str"="14.62500", "file path"=path "D:/Data/Ultrasound/LSCO/LSCO22__130814c/5_Cooling_2nd_try/September_2014/091814/14.62500K_500_2500_2.10000V_0.00000T_Sep18-2014__09-50-06_001_091814.bin", "last mod"=timestamp(3493893006 s since 1904-01-01), "file name str"="D:\\Data\\Ultrasound\\LSCO\\LSCO22__130814c\\5_Cooling_2nd_try\\September_2014\\091814\\14.62500K_500_2500_2.10000V_0.00000T_Sep18-2014__09-50-06_001_091814.bin", "mod time(min)"=58231550.1, "file format"=enum."binary", "power(V)"=2.1, "Magn Field(T) "=0.0}, {"temperature"=14.628, "temperature str"="14.62800", "file path"=path "D:/Data/Ultrasound/LSCO/LSCO22__130814c/5_Cooling_2nd_try/September_2014/091814/14.62800K_500_2500_2.10000V_0.00000T_Sep18-2014__09-51-26_001_091814.bin", "last mod"=timestamp(3493893086 s since 1904-01-01), "file name str"="D:\\Data\\Ultrasound\\LSCO\\LSCO22__130814c\\5_Cooling_2nd_try\\September_2014\\091814\\14.62800K_500_2500_2.10000V_0.00000T_Sep18-2014__09-51-26_001_091814.bin", "mod time(min)"=58231551.43333333, "file format"=enum."binary", "power(V)"=2.1, "Magn Field(T) "=0.0}, {"temperature"=14.63, "temperature str"="14.63000", "file path"=path "D:/Data/Ultrasound/LSCO/LSCO22__130814c/5_Cooling_2nd_try/September_2014/091814/14.63000K_500_2500_2.10000V_0.00000T_Sep18-2014__09-52-45_001_091814.bin", "last mod"=timestamp(3493893165 s since 1904-01-01), "file name str"="D:\\Data\\Ultrasound\\LSCO\\LSCO22__130814c\\5_Cooling_2nd_try\\September_2014\\091814\\14.63000K_500_2500_2.10000V_0.00000T_Sep18-2014__09-52-45_001_091814.bin", "mod time(min)"=58231552.75, "file format"=enum."binary", "power(V)"=2.1, "Magn Field(T) "=0.0}, {"temperature"=14.63, "temperature str"="14.63000", "file path"=path "D:/Data/Ultrasound/LSCO/LSCO22__130814c/5_Cooling_2nd_try/September_2014/091814/14.63000K_500_2500_2.10000V_0.00000T_Sep18-2014__09-54-04_001_091814.bin", "last mod"=timestamp(3493893244 s since 1904-01-01), "file name str"="D:\\Data\\Ultrasound\\LSCO\\LSCO22__130814c\\5_Cooling_2nd_try\\September_2014\\091814\\14.63000K_500_2500_2.10000V_0.00000T_Sep18-2014__09-54-04_001_091814.bin", "mod time(min)"=58231554.06666667, "file format"=enum."binary", "power(V)"=2.1, "Magn Field(T) "=0.0}, {"temperature"=14.635, "temperature str"="14.63500", "file path"=path "D:/Data/Ultrasound/LSCO/LSCO22__130814c/5_Cooling_2nd_try/September_2014/091814/14.63500K_500_2500_2.10000V_0.00000T_Sep18-2014__09-55-24_001_091814.bin", "last mod"=timestamp(3493893324 s since 1904-01-01), "file name str"="D:\\Data\\Ultrasound\\LSCO\\LSCO22__130814c\\5_Cooling_2nd_try\\September_2014\\091814\\14.63500K_500_2500_2.10000V_0.00000T_Sep18-2014__09-55-24_001_091814.bin", "mod time(min)"=58231555.4, "file format"=enum."binary", "power(V)"=2.1, "Magn Field(T) "=0.0}, {"temperature"=14.636, "temperature str"="14.63600", "file path"=path "D:/Data/Ultrasound/LSCO/LSCO22__130814c/5_Cooling_2nd_try/September_2014/091814/14.63600K_500_2500_2.10000V_0.00000T_Sep18-2014__09-56-43_001_091814.bin", "last mod"=timestamp(3493893403 s since 1904-01-01), "file name str"="D:\\Data\\Ultrasound\\LSCO\\LSCO22__130814c\\5_Cooling_2nd_try\\September_2014\\091814\\14.63600K_500_2500_2.10000V_0.00000T_Sep18-2014__09-56-43_001_091814.bin", "mod time(min)"=58231556.71666667, "file format"=enum."binary", "power(V)"=2.1, "Magn Field(T) "=0.0}, {"temperature"=14.637, "temperature str"="14.63700", "file path"=path "D:/Data/Ultrasound/LSCO/LSCO22__130814c/5_Cooling_2nd_try/September_2014/091814/14.63700K_500_2500_2.10000V_0.00000T_Sep18-2014__09-58-03_001_091814.bin", "last mod"=timestamp(3493893483 s since 1904-01-01), "file name str"="D:\\Data\\Ultrasound\\LSCO\\LSCO22__130814c\\5_Cooling_2nd_try\\September_2014\\091814\\14.63700K_500_2500_2.10000V_0.00000T_Sep18-2014__09-58-03_001_091814.bin", "mod time(min)"=58231558.05, 
